vi "TRAJECTORY_EXECUTE_SWERVE.vi"(6 "EnableClosedLoop":bool=TRUE, 7 "Orientation Dmd In":dbl, 8 "Init":bool, 9 "Reverse":bool, 10 "Follow Orientation":bool, 11 "Gyro Heading":dbl) -> (0 "AtReference":bool, 1 "OutputTRAJ_STATE":T2={"TimeSeconds"=0.0, "Velocity"=0.0, "Acceleration"=0.0, "POSE"={"TRANSLATION"={"X"=0.0, "Y"=0.0}, "ROTATION"={"VALUE"=0.0, "COS"=1.0, "SIN"=0.0}}, "Curvature"=0.0} {"POSE"."ROTATION"."SIN" format="%13.4f"; "POSE"."ROTATION"."COS" format="%13.4f"; "POSE"."ROTATION"."VALUE" format="%13.4f"; "POSE"."TRANSLATION"."Y" format="%14.3f"; "POSE"."TRANSLATION"."X" format="%14.3f"}, 2 "Error Pose":T3 {"ROTATION"."SIN" format="%13.4f"; "ROTATION"."COS" format="%13.4f"; "ROTATION"."VALUE" format="%13.4f"; "TRANSLATION"."Y" format="%14.3f"; "TRANSLATION"."X" format="%14.3f"}, 3 "Chassis Velocity Target":T1 {"vOmega" format="%10.3f"; "vY" format="%10.3f"; "vX" format="%10.3f"}, 5 "Orientation Target":dbl)   [LabVIEW 2019]
uses:
  <vilib>/Rock Robotics/WPI/ThirdParty/JAS_Junk/TrajLib/POSE2D.ctl
  <vilib>/Rock Robotics/WPI/ThirdParty/JAS_Junk/TrajLib/TRANSLATION2D.ctl
  <vilib>/Rock Robotics/WPI/ThirdParty/JAS_Junk/TrajLib/ROTATION2D.ctl
  <vilib>/Rock Robotics/WPI/ThirdParty/JAS_Junk/TrajLib/TRAJ_STATE.ctl
  <vilib>/Rock Robotics/WPI/ThirdParty/JAS_Junk/TrajLib/CHASSIS_SPEEDS.ctl
  <vilib>/Rock Robotics/WPI/ThirdParty/JAS_Junk/TrajLib/Translation_Create.vi
  <vilib>/Rock Robotics/WPI/ThirdParty/JAS_Junk/TrajLib/Rotation_UnaryMinus.vi
  <vilib>/Rock Robotics/WPI/ThirdParty/JAS_Junk/TrajLib/Rotation_RotateBy.vi
  <vilib>/Rock Robotics/WPI/ThirdParty/JAS_Junk/TrajLib/PIDController_Calculate_SP_PV.vi
  <vilib>/Rock Robotics/WPI/ThirdParty/JAS_Junk/TrajLib/PIDController_AtSetpoint.vi
  <vilib>/Rock Robotics/WPI/ThirdParty/JAS_Junk/TrajLib/PIDController_SetPID.vi
  <vilib>/Rock Robotics/WPI/ThirdParty/JAS_Junk/TrajLib/PIDController_SetIntegratorRange.vi
  <vilib>/Rock Robotics/WPI/ThirdParty/JAS_Junk/TrajLib/PIDController_SetTolerancePandV.vi
  <vilib>/Rock Robotics/WPI/ThirdParty/JAS_Junk/TrajLib/PIDController_DisableContinousInput.vi
  <vilib>/Rock Robotics/WPI/ThirdParty/JAS_Junk/TrajLib/PIDController_SetInputRange.vi
  <vilib>/Rock Robotics/WPI/ThirdParty/JAS_Junk/TrajLib/PIDController_EnableContinousInput.vi
  <vilib>/Rock Robotics/WPI/ThirdParty/JAS_Junk/TrajLib/PIDController_Reset.vi
  <vilib>/Rock Robotics/WPI/ThirdParty/JAS_Junk/TrajLib/PIDController_NewPeriod.vi
  <vilib>/Rock Robotics/WPI/ThirdParty/JAS_Junk/TrajLib/Rotation_GetCos.vi
  <vilib>/Rock Robotics/WPI/ThirdParty/JAS_Junk/TrajLib/Rotation_GetSin.vi
  <vilib>/Rock Robotics/WPI/ThirdParty/JAS_Junk/TrajLib/Rotation_CreateXY.vi
  <vilib>/Rock Robotics/WPI/ThirdParty/JAS_Junk/TrajLib/PIDController_SetSetpoint.vi
  <vilib>/Rock Robotics/WPI/ThirdParty/JAS_Junk/TrajLib/PIDController_Calculate_PV.vi
  <vilib>/Rock Robotics/SystemInterfaces/NetworkCommunication/NetComm_UsageReport_report.vi
  <vilib>/Rock Robotics/WPI/ThirdParty/JAS_Junk/TrajLib/Util_CalcDist.vi
  <vilib>/Rock Robotics/WPI/ThirdParty/JAS_Junk/TrajLib/PIDController_GetContinuousError.vi
  <vilib>/Rock Robotics/WPI/ThirdParty/JAS_Junk/TrajLib/Util_LibraryGlobals.vi
  <vilib>/Rock Robotics/WPI/ThirdParty/JAS_Junk/TrajLib/Trajectory_Library.lvlib
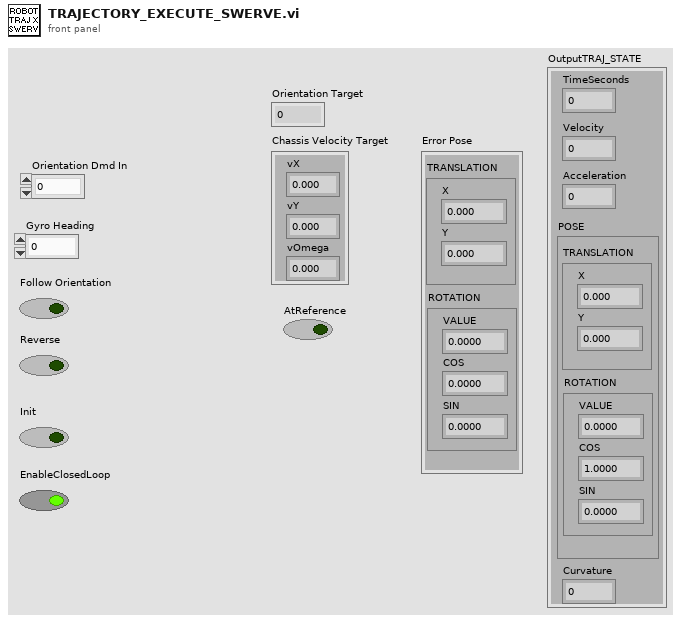
[diagram p1: front panel]
types:
  T1 = typedef "Trajectory_Library.lvlib/CHASSIS_SPEEDS.ctl" = cluster{"vX":dbl, "vY":dbl, "vOmega":dbl}
  T2 = typedef "Trajectory_Library.lvlib/TRAJ_STATE.ctl" = cluster{"TimeSeconds":dbl, "Velocity":dbl, "Acceleration":dbl, "POSE":T3, "Curvature":dbl}
  T3 = typedef "Trajectory_Library.lvlib/POSE2D.ctl" = cluster{"TRANSLATION":T4, "ROTATION":T5}
  T4 = typedef "Trajectory_Library.lvlib/TRANSLATION2D.ctl" = cluster{"X":dbl, "Y":dbl}
  T5 = typedef "Trajectory_Library.lvlib/ROTATION2D.ctl" = cluster{"VALUE":dbl, "COS":dbl, "SIN":dbl}
  T6 = typedef "Trajectory_Library.lvlib/SWERVE_DRIVE_KINEMATICS.ctl" = cluster{"NumModules":i32, "InverseKinematics":T7, "ForwardKinematics":T7, "Modules":T4[], "PrevCoR":T4}
  T7 = typedef "NI_Matrix.lvlib/RealMatrix.ctl" = dbl[][]
  T8 = typedef "Trajectory_Library.lvlib/SWERVE_DRIVE_ODOMETRY.ctl" = cluster{"POSE":T3, "GyroOffset":T5, "PreviousAngle":T5, "PrevTime":dbl}
  T9 = typedef "Trajectory_Library.lvlib/TRAJECTORY.ctl" = cluster{"TotalTImeSecs":dbl, "States":T2[]}
  T10 = typedef "Trajectory_Library.lvlib/SWERVE_DRIVE_MODULE_STATE.ctl" = cluster{"Speed":dbl, "Angle":T5}
  T11 = typedef "Trajectory_Library.lvlib/PID_TUNING.ctl" = cluster{"Kp":dbl, "Ki":dbl, "Kd":dbl, "MaximumIntegral":dbl, "MinimumIntegral":dbl}
  T12 = typedef "Trajectory_Library.lvlib/PID_ERROR_TOLERANCE.ctl" = cluster{"PositionTolerance":dbl, "VelocityTolerance":dbl}
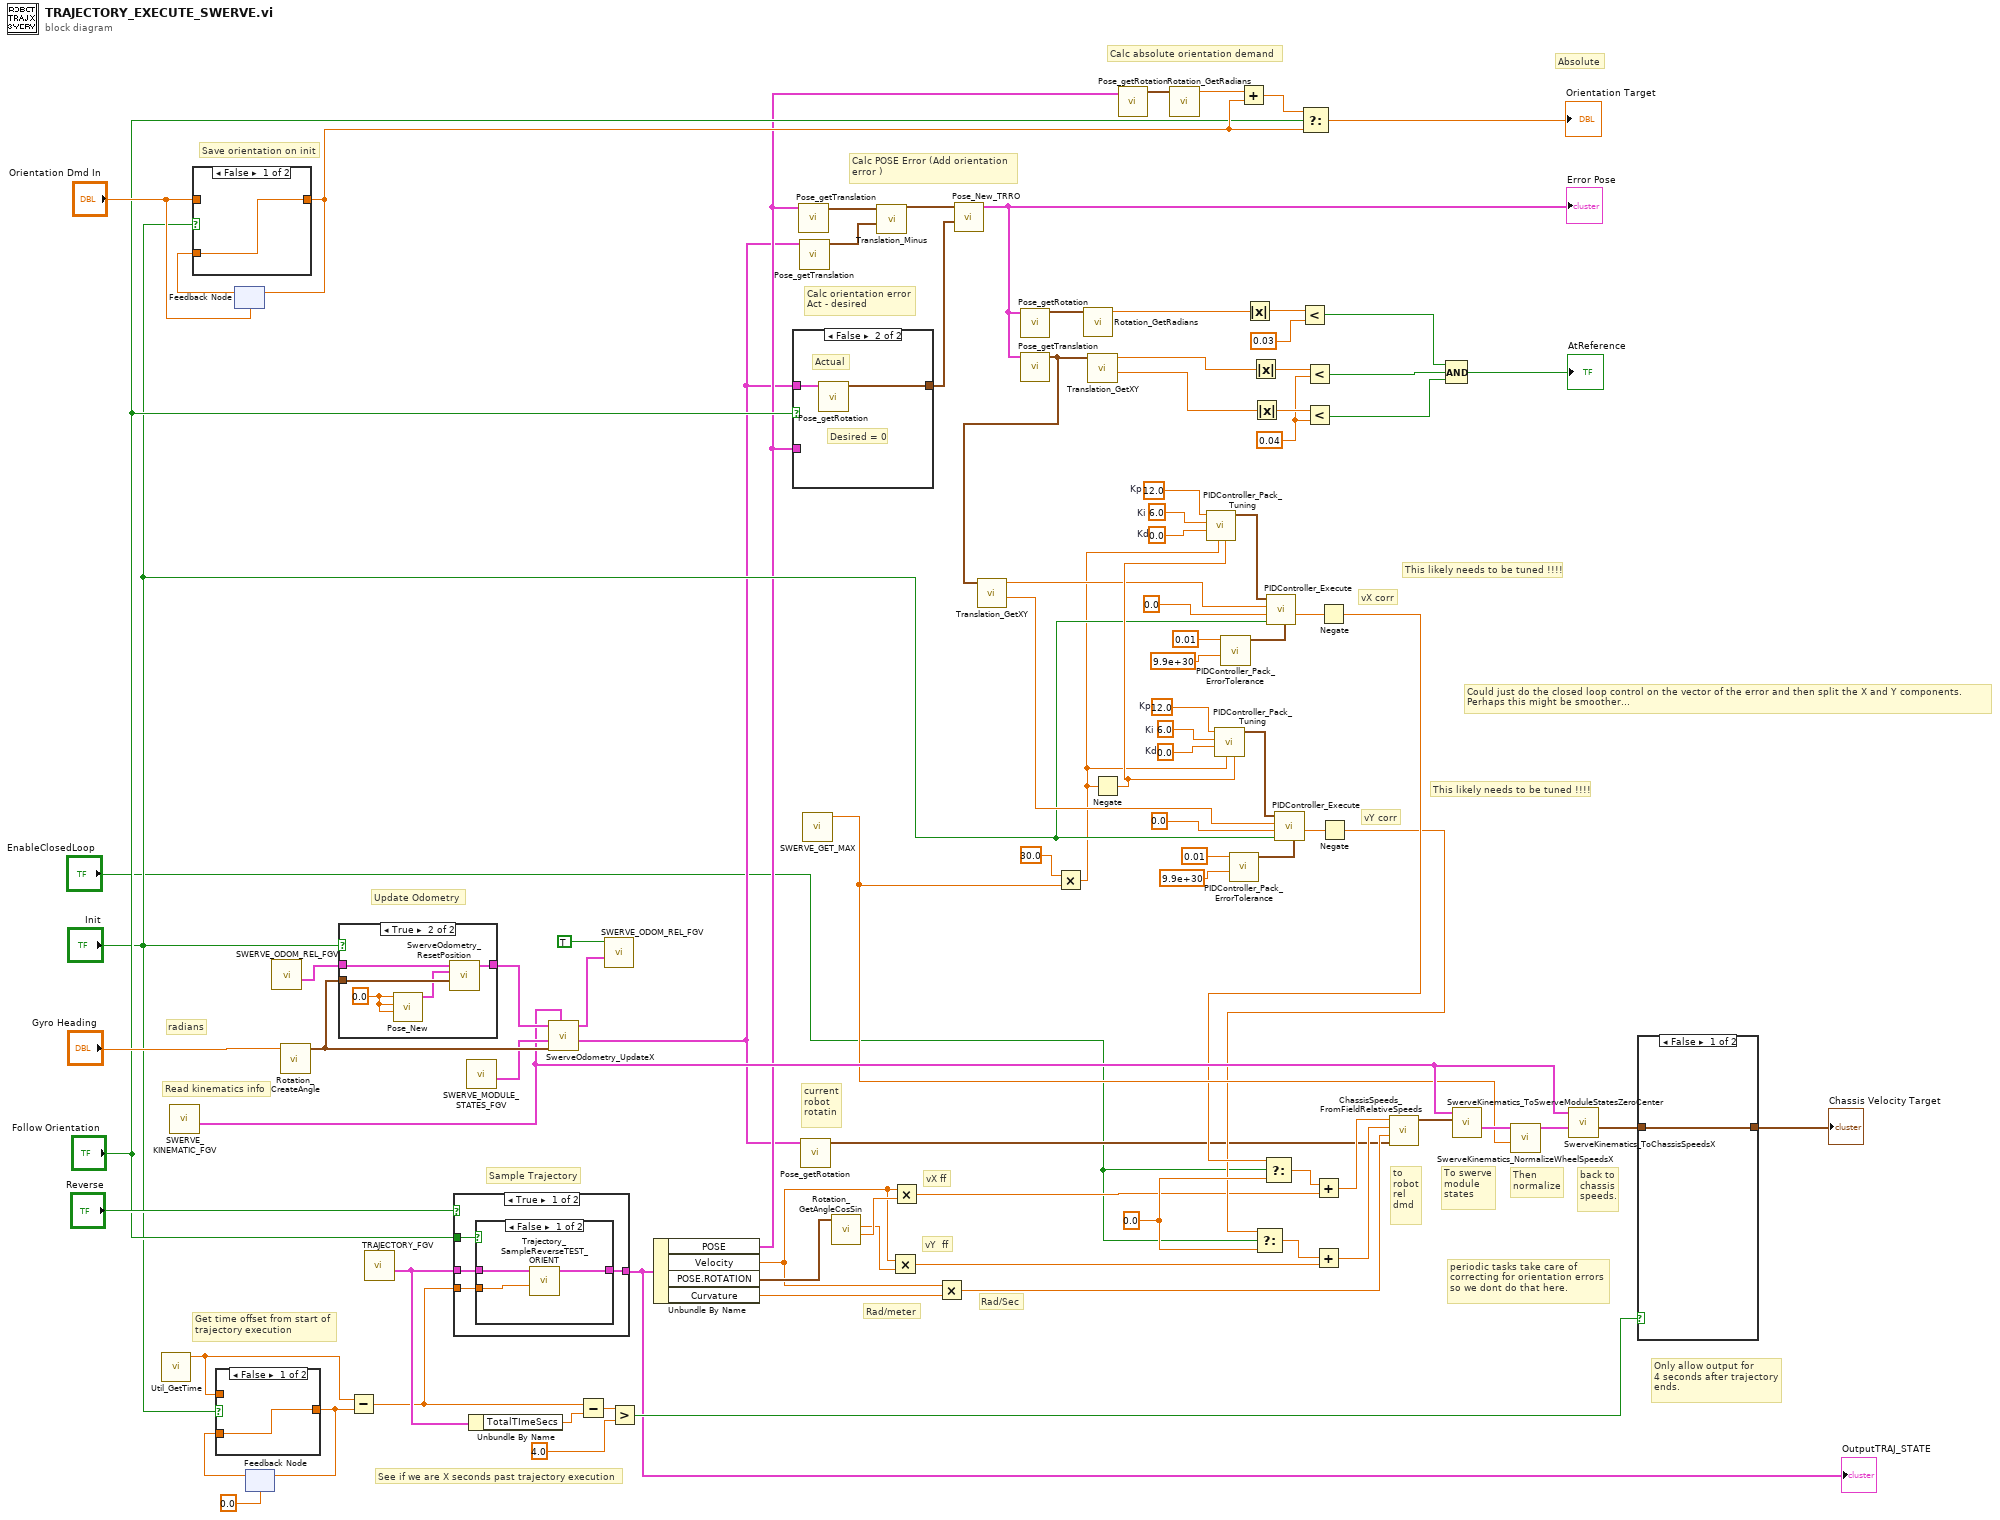
[diagram p0: block diagram]
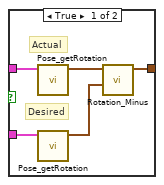
[diagram p2: hidden frame]
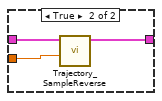
[diagram p3: hidden frame]
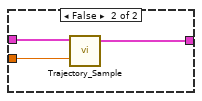
[diagram p4: hidden frame]
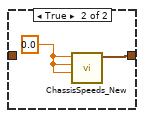
[diagram p7: hidden frame]
diagram:
  w33 = 0.0  # Kd
  w34 = 6.0  # Ki
  w35 = 12.0  # Kp
  w42 = 0.0  # Kd
  w43 = 6.0  # Ki
  w44 = 12.0  # Kp
  w53 = 0.0 ("f")
  w76 = 0.04
  # "to\nrobot\nrel\ndmd"
  # "This likely needs to be tuned !!!!"
  # "This likely needs to be tuned !!!!"
  # "Could just do the closed loop control on the vector of the error and then split the X and Y components.  \nPerhaps this might be smoother..."
  # "vY corr"
  # "vX corr"
  # "current\nrobot\nrotatin"
  # "vY  ff"
  # "vX ff"
  # "back to\nchassis\nspeeds."
  # "Then\nnormalize"
  # "To swerve\nmodule\nstates"
  # "Rad/Sec"
  # "Rad/meter"
  # "Calc POSE Error (Add orientation\nerror )"
  # "Calc orientation error\nAct - desired"
  # "Calc absolute orientation demand"
  # "Read kinematics info"
  # "Sample Trajectory"
  # "See if we are X seconds past trajectory execution"
  # "Get time offset from start of\ntrajectory execution"
  # "Save orientation on init"
  # "Absolute"
  # "Update Odometry"
  # "radians"
  # "periodic tasks take care of\ncorrecting for orientation errors\nso we dont do that here."
  # "Only allow output for\n4 seconds after trajectory\nends."
  n1 = call <vilib>:"Util_GetTime.vi"() -> ("FPGA_Time_Seconds"=w68:dbl)  [unwired: 10 in, 1 out]
  n2 = call "SWERVE_KINEMATIC_FGV.vi"() -> ("out SWERVE_DRIVE_KINEMATICS"=w69:T6)  [unwired: 11 in]
  n3 = feedback #1("Orientation Dmd In") -> (w66:dbl)
  n4 = case shown="False" "Init" {
    tunnel: "Orientation Dmd In" -> [_ w98]
    tunnel: [w97 w98] -> w63
    tunnel: w66 -> [w97 _]
    frame False {
    }
    frame True {
    }
  }
  n5 = feedback-in #1(w63) -> ()
  n6 = feedback #2(0.0 ("TIME")) -> (w95:dbl)
  n7 = case shown="False" "Init" {
    tunnel: [w99 w100] -> w94
    tunnel: w95 -> [w99 _]
    tunnel: w68 -> [_ w100]
    frame False {
    }
    frame True {
    }
  }
  n8 = feedback-in #2(w94) -> ()
  n9 = call "SWERVE_ODOM_REL_FGV.vi"() -> ("out SWERVE_DRIVE_ODOMETRY"=w86:T8)  [unwired: 11 in]
  n10 = call <vilib>:"Rotation_CreateAngle.vi"("Angle"="Gyro Heading") -> ("ROTATION"=w84:T5)  [unwired: 10 in]
  n11 = case shown="True" "Init" {
    tunnel: w86 -> [w101 w106]
    tunnel: [w101 w105] -> w85
    tunnel: w84 -> [_ w104]
    frame False {
    }
    frame True {
      w103 = 0.0 ("X")
      n12 = call <vilib>:"Pose_New.vi"("Heading"=w103, "Y"=w103, "X"=w103) -> ("out POSe"=w102:T3)  [unwired: 8 in]
      n13 = call <vilib>:"SwerveOdometry_ResetPosition.vi"("gyroAngle"=w104, "Pose"=w102, "in SWERVE_DRIVE_ODOMETRY"=w106) -> ("out SWERVE_DRIVE_ODOMETRY"=w105:T8)  [unwired: 8 in]
    }
  }
  n14 = Subtract(x=w68, y=w94) -> (x-y=w91:dbl)
  n15 = call "TRAJECTORY_FGV.vi"() -> ("outTRAJECTORY"=w93:T9)  [unwired: 11 in]
  n16 = case shown="True" "Reverse" {
    tunnel: w93 -> [w110 w119]
    tunnel: w91 -> [w108 w118]
    tunnel: [w109 w117] -> w81
    tunnel: "Follow Orientation" -> [w107 _]
    frame True {
      n17 = case shown="False" w107 {
        tunnel: w110 -> [w113 w116]
        tunnel: [w112 w115] -> w109
        tunnel: w108 -> [w111 w114]
        frame False {
          n18 = call "Trajectory_SampleReverseTEST_ORIENT.vi"("Time"=w111, "InputTRAJECTORY"=w113) -> ("OutputTRAJ_STATE"=w112:T2)  [unwired: 9 in]
        }
        frame True {
          n19 = call <vilib>:"Trajectory_SampleReverse.vi"("Time"=w114, "InputTRAJECTORY"=w116) -> ("OutputTRAJ_STATE"=w115:T2)  [unwired: 9 in]
        }
      }
    }
    frame False {
      n20 = call <vilib>:"Trajectory_Sample.vi"("Time"=w118, "InputTRAJECTORY"=w119) -> ("OutputTRAJ_STATE"=w117:T2)  [unwired: 9 in]
    }
  }
  "OutputTRAJ_STATE" <- w81
  n21 = call "SWERVE_MODULE_STATES_FGV.vi"() -> ("out Current Module States"=w82:T10[])  [unwired: 11 in]
  n22 = Unbundle By Name(w93) -> ("TotalTImeSecs"=w92:dbl)
  n23 = call <vilib>:"SwerveOdometry_UpdateX.vi"("SWERVE_DRIVE_KINEMATICS"=w69, "gyroAngle"=w84, "module States"=w82, "in SWERVE_DRIVE_ODOMETRY"=w85) -> ("robot POSE"=w5:T3, "out SWERVE_DRIVE_ODOMETRY"=w59:T8)  [unwired: 6 in]
  n24 = Subtract(x=w91, y=w92) -> (x-y=w90:dbl)
  n25 = call "SWERVE_ODOM_REL_FGV.vi"("in SWERVE_DRIVE_ODOMETRY"=w59, "WRITE"=TRUE) -> ()  [unwired: 9 in, 1 out]
  n26 = Greater?(x=w90, y=4.0) -> (0:w88:bool)
  n27 = Unbundle By Name(w81) -> ("POSE"=w6:T3, "Velocity"=w17:dbl, "POSE.ROTATION"=w20:T5, "Curvature"=w58:dbl)
  n28 = case shown="False" "Follow Orientation" {
    tunnel: w5 -> [w124 w126]
    tunnel: w6 -> [w123 _]
    tunnel: [w120 w125] -> w54
    frame True {
      # "Desired"
      # "Actual"
      n29 = call <vilib>:"Pose_getRotation.vi"("in POSE"=w124) -> ("out ROTATION"=w122:T5)  [unwired: 10 in]
      n30 = call <vilib>:"Pose_getRotation.vi"("in POSE"=w123) -> ("out ROTATION"=w121:T5)  [unwired: 10 in]
      n31 = call <vilib>:"Rotation_Minus.vi"("other ROTATION"=w121, "in ROTATION"=w122) -> ("out ROTATION"=w120:T5)  [unwired: 9 in]
    }
    frame False {
      # "Desired = 0"
      # "Actual"
      n32 = call <vilib>:"Pose_getRotation.vi"("in POSE"=w126) -> ("out ROTATION"=w125:T5)  [unwired: 10 in]
    }
  }
  n33 = call <vilib>:"Pose_getTranslation.vi"("in POSE"=w6) -> ("outTRANSLATION"=w4:T4)  [unwired: 10 in]
  n34 = call <vilib>:"Pose_getTranslation.vi"("in POSE"=w5) -> ("outTRANSLATION"=w3:T4)  [unwired: 10 in]
  n35 = call <vilib>:"Pose_getRotation.vi"("in POSE"=w5) -> ("out ROTATION"=w8:T5)  [unwired: 10 in]
  n36 = call "SWERVE_GET_MAX.vi"() -> ("Max Wheel Vel (Meter/Sec)"=w30:dbl)  [unwired: 10 in, 1 out]
  n37 = call <vilib>:"Rotation_GetAngleCosSin.vi"("in ROTATION"=w20) -> ("Cosine"=w19:dbl, "Sine"=w18:dbl)  [unwired: 8 in, 1 out]
  n38 = call <vilib>:"Translation_Minus.vi"("other Translation"=w3, "In Translation"=w4) -> ("Out Translation"=w2:T4)  [unwired: 9 in]
  n39 = Multiply(x=w17, y=w18) -> (x*y=w16:dbl)
  n40 = Multiply(x=w17, y=w19) -> (x*y=w15:dbl)
  n41 = Multiply(x=w17, y=w58) -> (x*y=w9:dbl)
  n42 = call <vilib>:"Pose_New_TRRO.vi"("ROTATION"=w54, "TRANSLATION"=w2) -> ("outPOSE"=w51:T3)  [unwired: 9 in]
  "Error Pose" <- w51
  n43 = call <vilib>:"Pose_getRotation.vi"("in POSE"=w51) -> ("out ROTATION"=w48:T5)  [unwired: 10 in]
  n44 = call <vilib>:"Pose_getTranslation.vi"("in POSE"=w51) -> ("outTRANSLATION"=w14:T4)  [unwired: 10 in]
  n45 = call <vilib>:"Translation_GetXY.vi"("In Translation"=w14) -> ("Y"=w27:dbl, "X"=w28:dbl)  [unwired: 9 in]
  n46 = Multiply(x=30.0, y=w30) -> (x*y=w21:dbl)
  n47 = call <vilib>:"Rotation_GetRadians.vi"("in ROTATION"=w48) -> ("AngleRadians"=w50:dbl)  [unwired: 10 in]
  n48 = call <vilib>:"Translation_GetXY.vi"("In Translation"=w14) -> ("Y"=w49:dbl, "X"=w52:dbl)  [unwired: 9 in]
  n49 = Negate(x=w21) -> (-x=w29:dbl)
  n50 = call <vilib>:"Pose_getRotation.vi"("in POSE"=w6) -> ("out ROTATION"=w64:T5)  [unwired: 10 in]
  n51 = call <vilib>:"Rotation_GetRadians.vi"("in ROTATION"=w64) -> ("AngleRadians"=w62:dbl)  [unwired: 10 in]
  n52 = call <vilib>:"PIDController_Pack_Tuning.vi"("MinimumIntegral"=w29, "MaximumIntegral"=w21, "Kd"=w42, "Ki"=w43, "Kp"=w44) -> ("PID Tuning"=w47:T11)  [unwired: 6 in]
  n53 = call <vilib>:"PIDController_Pack_Tuning.vi"("MinimumIntegral"=w29, "MaximumIntegral"=w21, "Kd"=w33, "Ki"=w34, "Kp"=w35) -> ("PID Tuning"=w38:T11)  [unwired: 6 in]
  n54 = call <vilib>:"PIDController_Pack_ErrorTolerance.vi"("VelocityTolerance"=9.9e+30, "PositionTolerance"=0.01) -> ("PID Error Tolerance"=w45:T12)  [unwired: 9 in]
  n55 = call <vilib>:"PIDController_Pack_ErrorTolerance.vi"("VelocityTolerance"=9.9e+30, "PositionTolerance"=0.01) -> ("PID Error Tolerance"=w36:T12)  [unwired: 9 in]
  n56 = Add(x=w62, y=w63) -> (x+y=w61:dbl)
  n57 = Absolute Value(x=w50) -> (abs(x)=w80:dbl)
  n58 = Absolute Value(x=w52) -> (abs(x)=w79:dbl)
  n59 = Absolute Value(x=w49) -> (abs(x)=w78:dbl)
  n60 = call <vilib>:"PIDController_Execute.vi"("PID Error Tolerance"=w45, "Reset"="Init", "SP-SetPoint"=0.0, "PV-Measurement"=w28, "PID Tuning"=w47) -> ("CO-ControlOutput"=w26:dbl)  [unwired: 4 in, 2 out]
  n61 = call <vilib>:"PIDController_Execute.vi"("PID Error Tolerance"=w36, "Reset"="Init", "SP-SetPoint"=0.0, "PV-Measurement"=w27, "PID Tuning"=w38) -> ("CO-ControlOutput"=w25:dbl)  [unwired: 4 in, 2 out]
  n62 = Less?(x=w80, y=0.03) -> (x < y?=w75:bool)
  n63 = Select(t=w61, s="Follow Orientation", f=w63) -> (s? t:f=→"Orientation Target":dbl)
  n64 = Less?(x=w79, y=w76) -> (x < y?=w74:bool)
  n65 = Less?(x=w78, y=w76) -> (x < y?=w73:bool)
  n66 = Negate(x=w26) -> (-x=w24:dbl)
  n67 = Select(t=w24, s="EnableClosedLoop", f=w53) -> (s? t:f=w13:dbl)
  n68 = Add(x=w13, y=w15) -> (x+y=w11:dbl)
  n69 = Negate(x=w25) -> (-x=w23:dbl)
  n70 = Select(t=w23, s="EnableClosedLoop", f=w53) -> (s? t:f=w12:dbl)
  n71 = Add(x=w12, y=w16) -> (x+y=w10:dbl)
  n72 = call <vilib>:"ChassisSpeeds_FromFieldRelativeSpeeds.vi"("RobotAngle"=w8, "Omega"=w9, "vY"=w10, "vX"=w11) -> ("CHASSIS"=w7:T1)  [unwired: 7 in]
  n73 = Compound Arithmetic op=AND(w75, w74, w73) -> (→"AtReference":bool)
  n74 = call <vilib>:"SwerveKinematics_ToSwerveModuleStatesZeroCenter.vi"("ChassisSpeeds"=w7, "in SWERVE_DRIVE_KINEMATICS"=w69) -> ("ModuleStates"=w71:T10[])  [unwired: 8 in, 1 out]
  n75 = call <vilib>:"SwerveKinematics_NormalizeWheelSpeedsX.vi"("AttainableMaxSpeed"=w30, "in WheelStates"=w71) -> ("out WheelStates"=w70:T10[])  [unwired: 9 in]
  n76 = call <vilib>:"SwerveKinematics_ToChassisSpeedsX.vi"("WheelStates"=w70, "in SWERVE_DRIVE_KINEMATICS"=w69) -> ("Chassis Speed"=w56:T1)  [unwired: 9 in]
  n77 = case shown="False" w88 {
    tunnel: w56 -> [w127 _]
    tunnel: [w127 w128] -> w55
    frame False {
    }
    frame True {
      w129 = 0.0 ("vX")
      n78 = call <vilib>:"ChassisSpeeds_New.vi"("vAngular"=w129, "vY"=w129, "vX"=w129) -> ("CHASSIS"=w128:T1)  [unwired: 8 in]
    }
  }
  "Chassis Velocity Target" <- w55
